vi "comms_Serial_Read_Packet.vi"(8 "error in":errorcluster, 11 "VISA resource in":refnum<visa-resource-name>) -> (0 "error out":errorcluster, 1 "Bytes_In_Buffer":u32, 2 "Data Out":string, 3 "VISA resource Out":refnum<visa-resource-name>)   [LabVIEW 2016]
panel:
  in  "Pkt Offset":i32=6
  out "Seek Its":i32
  out "Valid Packet?":bool
  # "s"
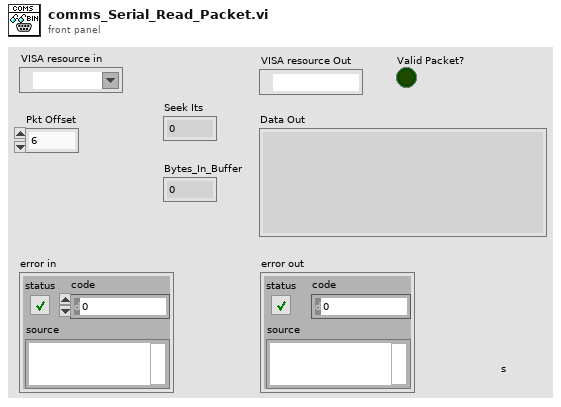
[diagram p1: front panel]
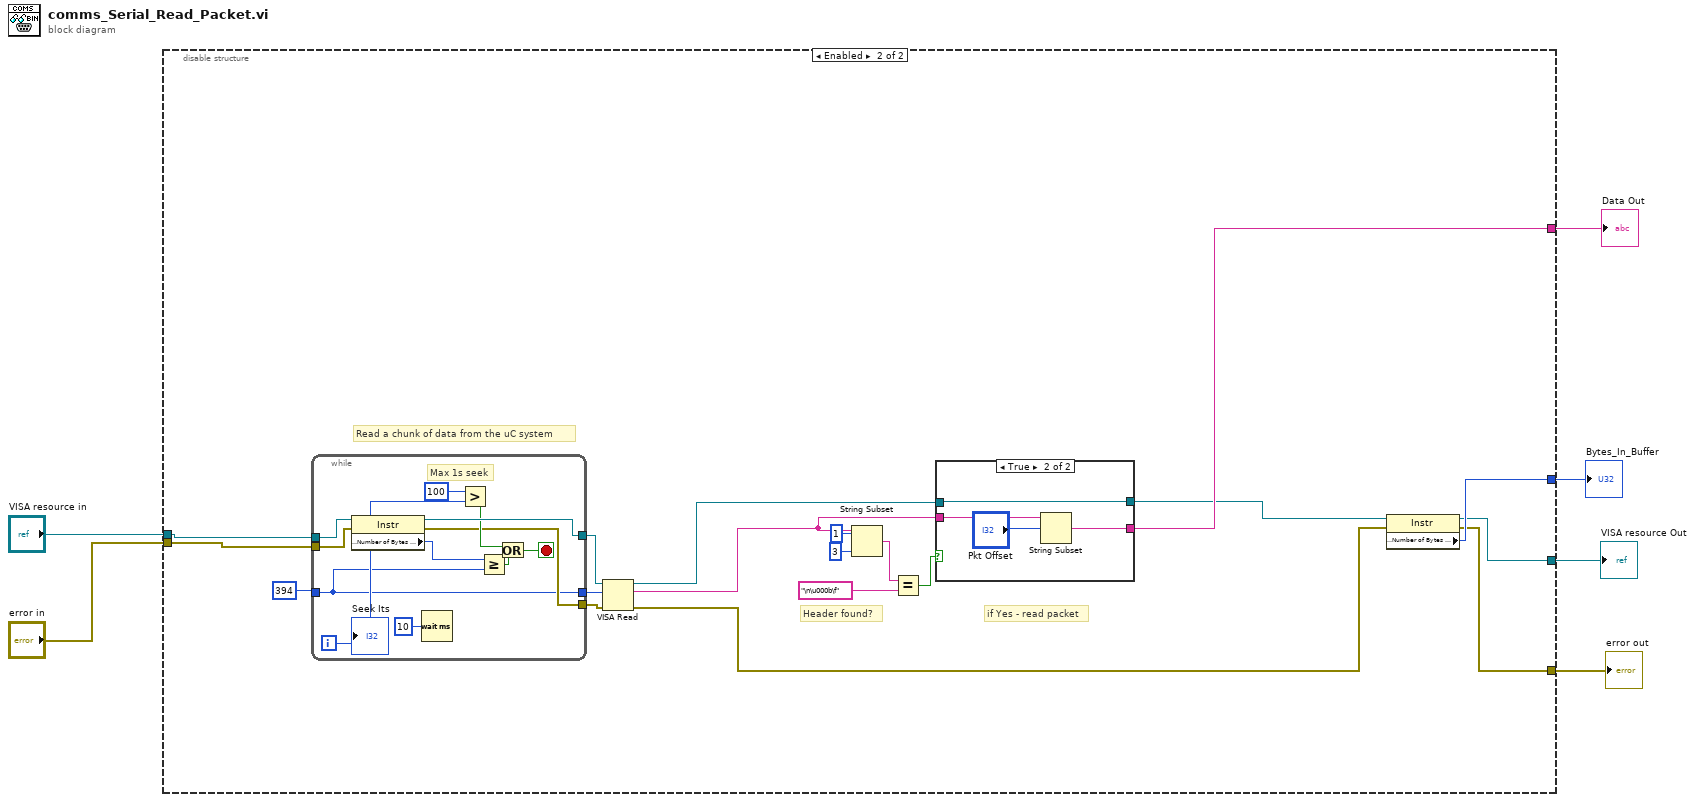
[diagram p0: block diagram]
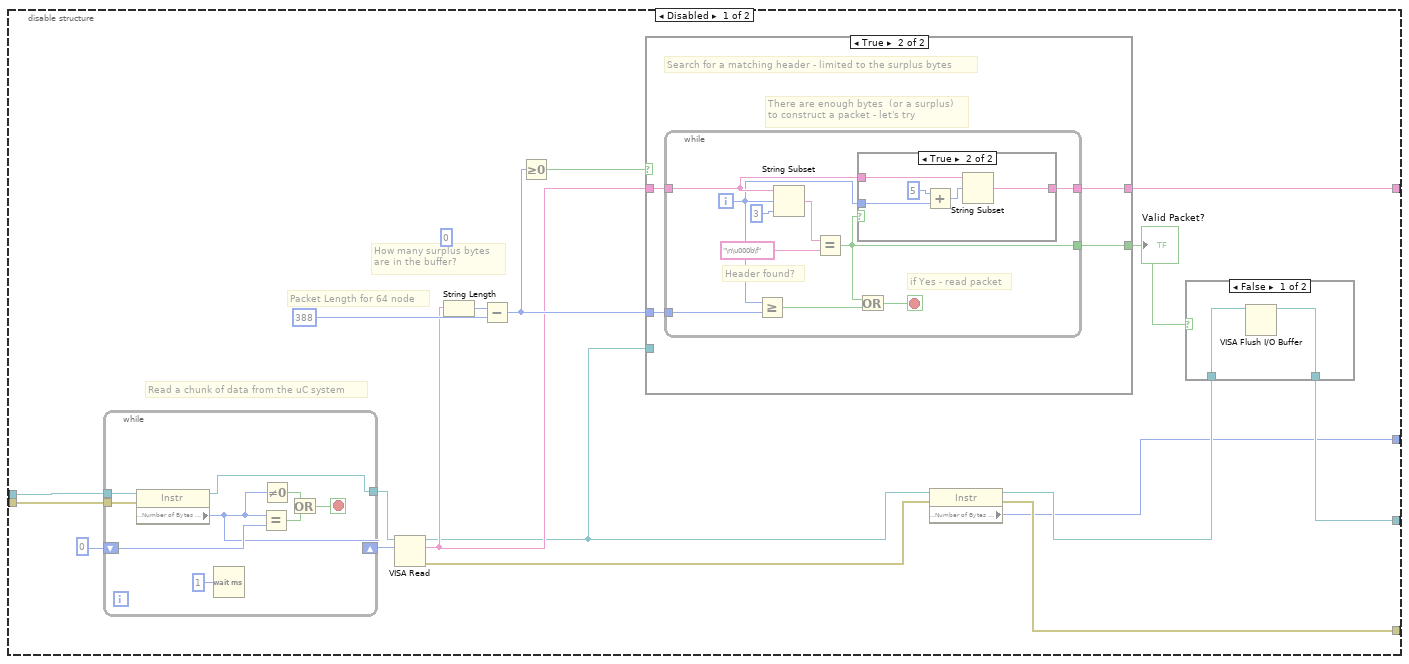
[diagram p2: hidden frame]
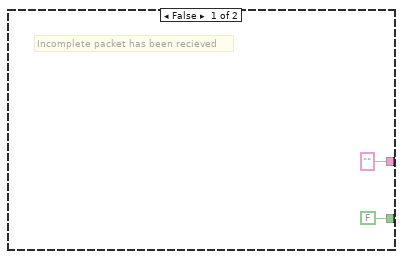
[diagram p4: hidden frame]
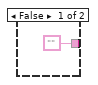
[diagram p5: hidden frame]
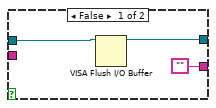
[diagram p6: hidden frame]
diagram:
  n1 = disable-structure shown="Enabled" {
    disable-tunnel: "VISA resource in" -> [w24 w74]
    disable-tunnel: "error in" -> [w20 w73]
    disable-tunnel: [w14 w66] -> w4
    disable-tunnel: [w13 w63] -> w3
    disable-tunnel: [w9 w60] -> w2
    disable-tunnel: [w7 w64] -> w1
    frame Disabled {
      (unwired) 0 ("length")
      # "Read a chunk of data from the uC system"
      # "Packet Length for 64 node"
      # "How many surplus bytes\nare in the buffer?"
      n2 = while {
        tunnel: w24 -> [w58]
        shift-right: [w51] -> w22
        shift-left: u32 0 ("byte count") -> [w56]
        tunnel: [w52] -> w23
        tunnel: w20 -> [w50]
        stop <- w53 stop-if-true
        n3 = property class="Instr"(reference=w58, error in=w50) -> (reference out=w52:refnum<visa-resource-name>, "Serial Settings:Number of Bytes at Serial Port"=w51:u32)  [unwired: 1 out]
        n4 = Wait (ms)(milliseconds to wait=u32 1) -> ()  [unwired: 1 out]
        n5 = Equal?(x=w51, y=w56) -> (x = y?=w54:bool)
        n6 = Not Equal To 0?(x=w51) -> (x != 0?=w55:bool)
        n7 = Or(x=w55, y=w54) -> (x .or. y?=w53:bool)
      }
      n8 = VISA Read(VISA resource name=w23, byte count=w22) -> (VISA resource name out=w11:refnum<visa-resource-name>, read buffer=w15:string, error out=w10:errorcluster)  [unwired: 1 in, 1 out]
      n9 = String Length(string=w15) -> (length=w19:i32)
      n10 = Subtract(x=w19, y=388 ("byte count")) -> (x-y=w17:i32)
      n11 = Greater Or Equal To 0?(x=w17) -> (x >= 0?=w18:bool)
      n12 = case shown="True" w18 {
        tunnel: w15 -> [_ w33]
        tunnel: ["" ("Data Out") w30] -> w14
        tunnel: w17 -> [_ w32]
        tunnel: [FALSE w31] -> w12
        tunnel: w11 -> [_ _]
        frame False {
          # "Incomplete packet has been recieved"
        }
        frame True {
          # "Search for a matching header - limited to the surplus bytes"
          # "There are enough bytes  (or a surplus)\nto construct a packet - let's try"
          n13 = while {
            tunnel: w33 -> [w35]
            tunnel: w32 -> [w42]
            tunnel: [w37] -> w31
            tunnel: [w36] -> w30
            i -> [w34]
            stop <- w41 stop-if-true
            # "if Yes - read packet"
            # "Header found?"
            n14 = Greater Or Equal?(x=w34, y=w42) -> (x >= y?=w40:bool)
            n15 = String Subset(string=w35, offset (0)=w34, length (rest)=3 ("length (rest)")) -> (substring=w39:string)
            n16 = Equal?(x=w39, y="\n\u000b\f") -> (x = y?=w37:bool)
            n17 = case shown="True" w37 {
              tunnel: ["" w49] -> w36
              tunnel: w35 -> [_ w48]
              tunnel: w34 -> [_ w46]
              frame False {
              }
              frame True {
                n18 = Add(x=5 ("length (rest)"), y=w46) -> (x+y=w47:i32)
                n19 = String Subset(string=w48, offset (0)=w47) -> (substring=w49:string)  [unwired: 1 in]
              }
            }
            n20 = Or(x=w37, y=w40) -> (x .or. y?=w41:bool)
          }
        }
      }
      "Valid Packet?" <- w12
      n21 = property class="Instr"(reference=w11, error in=w10) -> (reference out=w8:refnum<visa-resource-name>, error out=w9:errorcluster, "Serial Settings:Number of Bytes at Serial Port"=w7:u32)
      n22 = case shown="False" w12 {
        tunnel: w8 -> [w26 w27]
        tunnel: [w25 w27] -> w13
        frame False {
          n23 = VISA Flush I/O Buffer(VISA resource name=w26) -> (VISA resource name out=w25:refnum<visa-resource-name>)  [unwired: 2 in, 1 out]
        }
        frame True {
        }
      }
    }
    frame Enabled {
      # "if Yes - read packet"
      # "Header found?"
      # "Read a chunk of data from the uC system"
      n24 = while {
        tunnel: w74 -> [w96]
        tunnel: [w92] -> w77
        tunnel: w73 -> [w90]
        tunnel: [w86] -> w65
        tunnel: u32 394 ("byte count") -> [w85]
        tunnel: [w85] -> w76
        i -> [w88]
        stop <- w93 stop-if-true
        # "Max 1s seek"
        n25 = property class="Instr"(reference=w96, error in=w90) -> (reference out=w92:refnum<visa-resource-name>, error out=w86:errorcluster, "Serial Settings:Number of Bytes at Serial Port"=w91:u32)
        n26 = Wait (ms)(milliseconds to wait=u32 10) -> ()  [unwired: 1 out]
        n27 = Greater?(x=100, y=w88) -> (0:w89:bool)
        n28 = Greater Or Equal?(x=w91, y=w85) -> (x >= y?=w94:bool)
        n29 = Or(x=w89, y=w94) -> (x .or. y?=w93:bool)
        "Seek Its" <- w88
      }
      n30 = VISA Read(VISA resource name=w77, byte count=w76, error in (no error)=w65) -> (VISA resource name out=w67:refnum<visa-resource-name>, read buffer=w72:string, error out=w61:errorcluster)  [unwired: 1 out]
      n31 = String Subset(string=w72, offset (0)=1, length (rest)=3 ("length (rest)")) -> (substring=w70:string)
      n32 = Equal?(x=w70, y="\n\u000b\f") -> (x = y?=w68:bool)
      n33 = case shown="True" w68 {
        tunnel: ["" w84] -> w66
        tunnel: w72 -> [_ w83]
        tunnel: w67 -> [w79 w82]
        tunnel: [w78 w82] -> w62
        frame False {
          n34 = VISA Flush I/O Buffer(VISA resource name=w79) -> (VISA resource name out=w78:refnum<visa-resource-name>)  [unwired: 2 in, 1 out]
        }
        frame True {
          n35 = String Subset(string=w83, offset (0)="Pkt Offset") -> (substring=w84:string)  [unwired: 1 in]
        }
      }
      n36 = property class="Instr"(reference=w62, error in=w61) -> (reference out=w63:refnum<visa-resource-name>, error out=w60:errorcluster, "Serial Settings:Number of Bytes at Serial Port"=w64:u32)
    }
  }
  "VISA resource Out" <- w3
  "error out" <- w2
  "Data Out" <- w4
  "Bytes_In_Buffer" <- w1
